vi "2.2.vi"() -> ()   [LabVIEW 2020]
panel:
  out "Array":dbl[](array[numeric])
  out "Waveform Chart":dbl[](graph)
  out "appended array":dbl[][](array[numeric])
  out "Farenheit 2":dbl[](array[numeric])
  out "min value":dbl
  out "max value":dbl
  out "Celcius rand":dbl[](array[numeric])
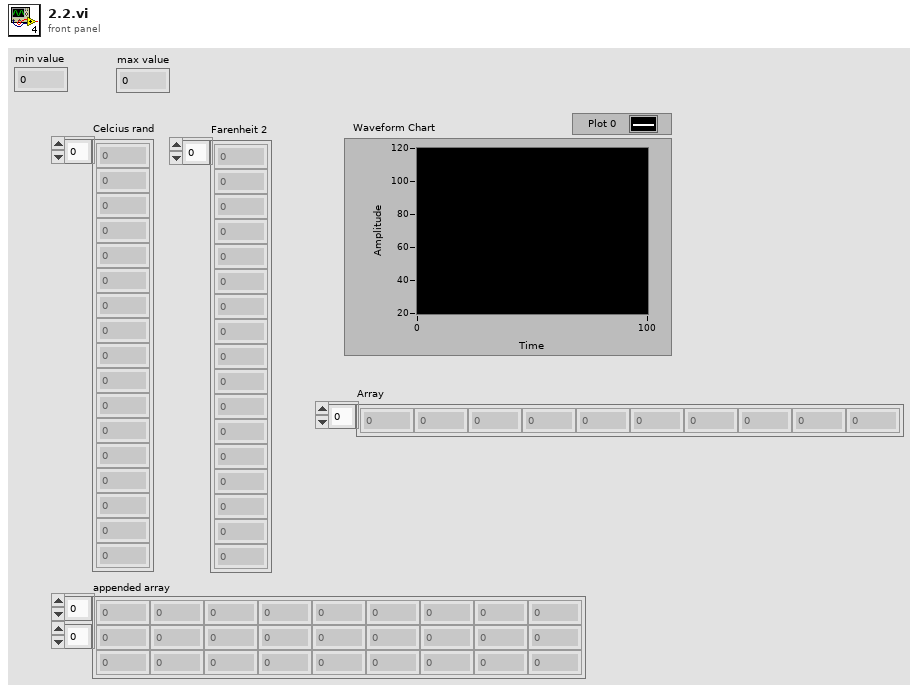
[diagram p1: front panel]
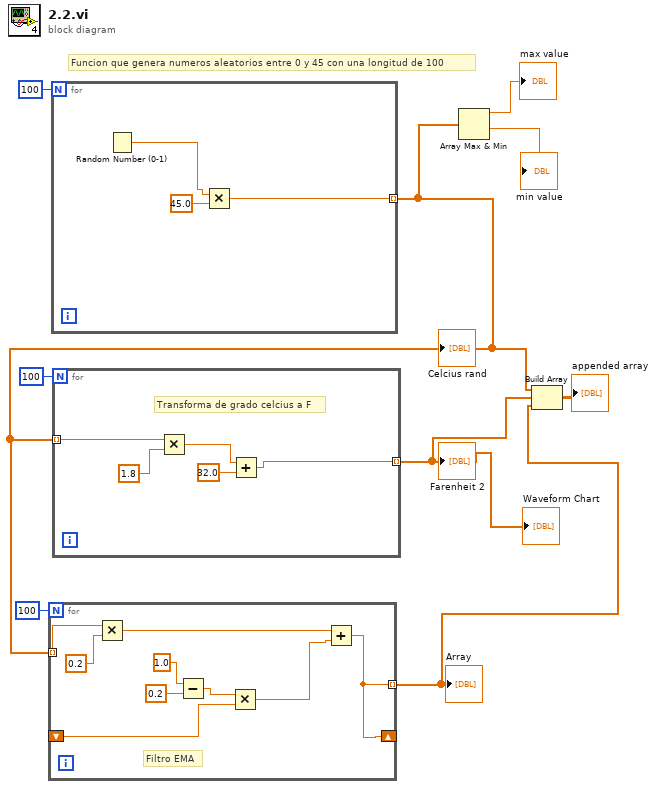
[diagram p0: block diagram]
diagram:
  # "Funcion que genera numeros aleatorios entre 0 y 45 con una longitud de 100"
  n1 = for {
    N: 100 -> [_]
    tunnel: [w10] -> w3 mode=indexing
    n2 = Random Number (0-1)() -> (number: 0 to 1=w11:dbl)
    n3 = Multiply(x=w11, y=45.0) -> (x*y=w10:dbl)
  }
  "Celcius rand" <- w3
  n4 = for {
    N: 100 -> [_]
    tunnel: w3 -> [w21] mode=indexing
    shift-right: [w13] -> _
    shift-left: _ -> [w15]
    tunnel: [w13] -> w1 mode=indexing
    # "Filtro EMA"
    n5 = Multiply(x=w21, y=0.2) -> (x*y=w19:dbl)
    n6 = Subtract(x=1.0, y=0.2) -> (x-y=w16:dbl)
    n7 = Multiply(x=w16, y=w15) -> (x*y=w14:dbl)
    n8 = Add(x=w19, y=w14) -> (x+y=w13:dbl)
  }
  "Array" <- w1
  n9 = for {
    N: 100 -> [_]
    tunnel: w3 -> [w26] mode=indexing
    tunnel: [w22] -> w4 mode=indexing
    # "Transforma de grado celcius a F"
    n10 = Multiply(x=w26, y=1.8) -> (x*y=w24:dbl)
    n11 = Add(x=w24, y=32.0) -> (x+y=w22:dbl)
  }
  "Farenheit 2" <- w4
  "Waveform Chart" <- w4
  n12 = Array Max & Min(array=w3) -> (max value=→"max value":dbl, min value=→"min value":dbl)  [unwired: 2 out]
  n13 = Build Array(w3, w4, w1) -> (→"appended array":dbl[][])
